vi "GLV_StreamToDisk.vi"(8 "error in":errorcluster, 9 "chunk size (bytes)":i32=65000, 10 "file size (GBytes)":dbl=5.0, 11 "filename":path=path "C:/big.bin") -> (0 "error out":errorcluster)   [LabVIEW 2014]
uses:
  Time/Timer_Global_Action_Control.ctl
panel:
  in  "Binary (t) / Text (f)":bool=TRUE
  out "Total (sec)":dbl
  out "Array":dbl[](array[numeric])
  out "progress":dbl(slide)=1.000003731250763 scale=0.0..1.0
  in  "stop":bool
  # "2,119GB 139,735sec %.6f string\n5GB 7,31sec"
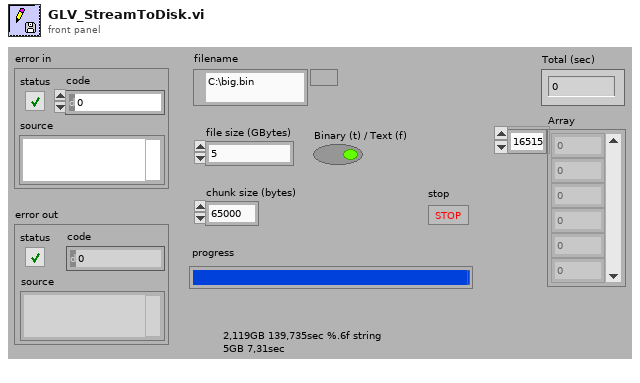
[diagram p1: front panel]
types:
  T1 = typedef "Timer_Global_Action_Control.ctl" = enum16{"Init", "Set", "Get", "Update", "Clear"}
  T2 = enum16{"open", "open or create", "create or replace", "create", "open (read only)"}
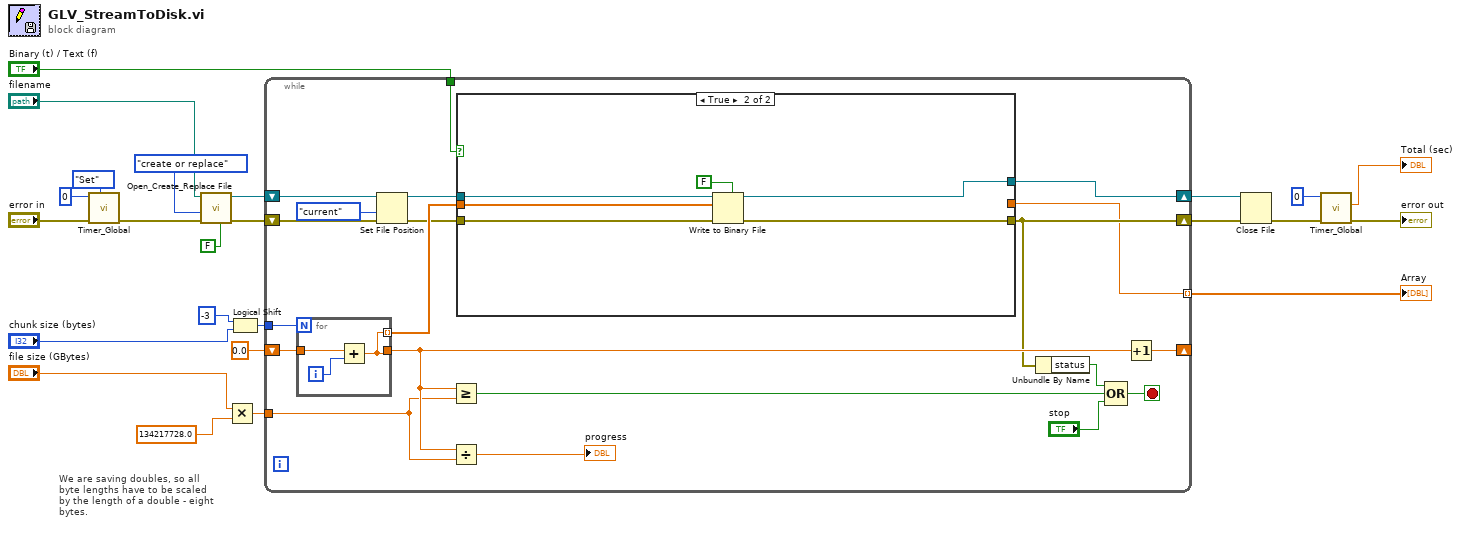
[diagram p0: block diagram]
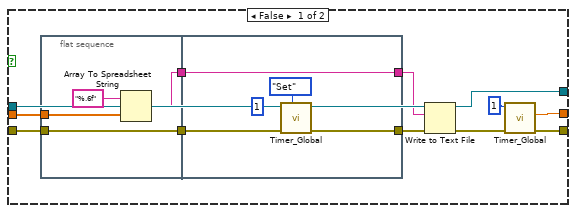
[diagram p2: hidden frame]
diagram:
  # "We are saving doubles, so all\nbyte lengths have to be scaled\nby the length of a double - eight\nbytes."
  n1 = call "Timer_Global.vi"("Timer Action (Get) (In)"=Timer_Global_Action_Control."Set", "Error In"="error in", "Timer ID (0) (In)"=0) -> ("Error Out"=w9:errorcluster)  [unwired: 6 in, 2 out]
  n2 = call <vilib>:"Open_Create_Replace File.vi"("advisory dialog? (display:T)"=FALSE, "error in (no error)"=w9, "function (open:0)"=T2."create or replace", "file path"="filename") -> ("error out"=w23:errorcluster, "refnum"=w15:refnum<file>)  [unwired: 4 in, 2 out]
  n3 = Multiply(x="file size (GBytes)", y=134217728.0) -> (x*y=w16:dbl)
  n4 = Logical Shift(y=-3, x="chunk size (bytes)") -> (x << y=w18:i32)
  n5 = while {
    shift-right: [w27] -> w14
    shift-left: w23 -> [w40]
    tunnel: w18 -> [w44]
    shift-right: [w30] -> _
    shift-left: 0.0 -> [w43]
    tunnel: w16 -> [w31]
    shift-right: [w38] -> w13
    shift-left: w15 -> [w39]
    tunnel: [w26] -> w3 mode=indexing
    tunnel: "Binary (t) / Text (f)" -> [w25]
    stop <- w36 stop-if-true
    n6 = for {
      N: w44 -> [_]
      tunnel: w43 -> [w74]
      tunnel: [w72] -> w32
      tunnel: [w72] -> w41 mode=indexing
      i -> [w73]
      n7 = Add(x=w74, y=w73) -> (x+y=w72:dbl)
    }
    n8 = Set File Position(refnum=w39, from (0:start)=enum16{"start", "end", "current"}."current" ("pos mode (0:2)"), error in=w40) -> (refnum out=w29:refnum<file>, error out=w28:errorcluster)  [unwired: 1 in]
    n9 = Greater Or Equal?(x=w32, y=w31) -> (x >= y?=w42:bool)
    n10 = Divide(x=w32, y=w31) -> (x/y=→"progress":dbl)
    n11 = case shown="True" w25 {
      tunnel: w41 -> [w54 w71]
      tunnel: [w56 w70] -> w38
      tunnel: w29 -> [w55 w69]
      tunnel: w28 -> [w50 w68]
      tunnel: [w46 w66] -> w27
      tunnel: [w45 _] -> w26
      frame False {
        n12 = flat-sequence {
          tunnel: w54 -> [w60]
          tunnel: [w59] -> w52
          tunnel: [w58] -> w51
          tunnel: w50 -> [w58]
          tunnel: [w65] -> w53
          tunnel: w52 -> [w65]
          tunnel: w51 -> [w62]
          tunnel: [w61] -> w49
          frame #0 {
            n13 = Array To Spreadsheet String(array=w60, 3:"%.6f" ("format string")) -> (spreadsheet string=w59:string)  [unwired: 1 in]
          }
          frame #1 {
            n14 = call "Timer_Global.vi"("Timer Action (Get) (In)"=Timer_Global_Action_Control."Set", "Error In"=w62, "Timer ID (0) (In)"=1) -> ("Error Out"=w61:errorcluster)  [unwired: 6 in, 2 out]
          }
        }
        n15 = Write to Text File(file (use dialog)=w55, text=w53, error in=w49) -> (refnum out=w56:refnum<file>, error out=w47:errorcluster)  [unwired: 1 in, 1 out]
        n16 = call "Timer_Global.vi"("Error In"=w47, "Timer ID (0) (In)"=1) -> ("Error Out"=w46:errorcluster, "Time Difference"=w45:dbl)  [unwired: 7 in, 1 out]
      }
      frame True {
        n17 = Write to Binary File(file (use dialog)=w69, data=w71, error in=w68, 5:FALSE ("prepend array or string size? (T)")) -> (refnum out=w70:refnum<file>, error out=w66:errorcluster)  [unwired: 2 in, 1 out]
      }
    }
    n18 = Unbundle By Name(w27) -> ("status"=w34:bool)
    n19 = Compound Arithmetic op=OR(w34, w42, "stop") -> (w36:bool)
    n20 = Increment(x=w32) -> (x+1=w30:dbl)
  }
  "Array" <- w3
  n21 = Close File(refnum=w13, error in=w14) -> (error out=w5:errorcluster)  [unwired: 1 out]
  n22 = call "Timer_Global.vi"("Error In"=w5, "Timer ID (0) (In)"=0) -> ("Error Out"=→"error out":errorcluster, "Time Difference"=→"Total (sec)":dbl)  [unwired: 7 in, 1 out]
